vi "SetTriggerPulseWidth.vi"(8 "Error In":errorcluster, 9 "Pulse Width (sec)":dbl, 10 "Line (1-14)":u8=1 min=1 max=14 step=1, 11 "Keithley 2602 In":refnum<visa-resource-name>) -> (0 "Error Out":errorcluster, 3 "Keithley 2602 Out":refnum<visa-resource-name>)   [LabVIEW 2012, in "Keithley-2602.lvlib"]
uses:
  Keithley-2602.lvlib
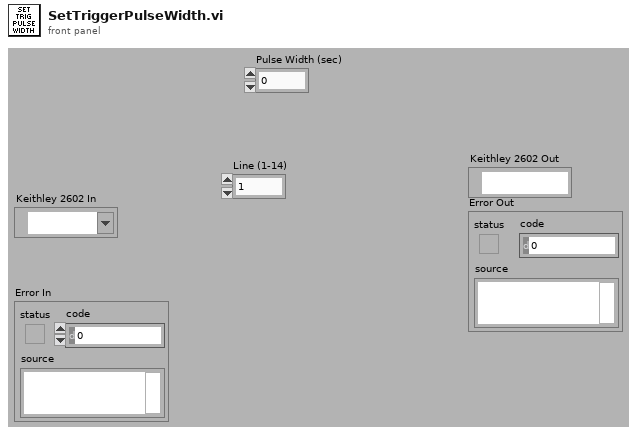
[diagram p1: front panel]
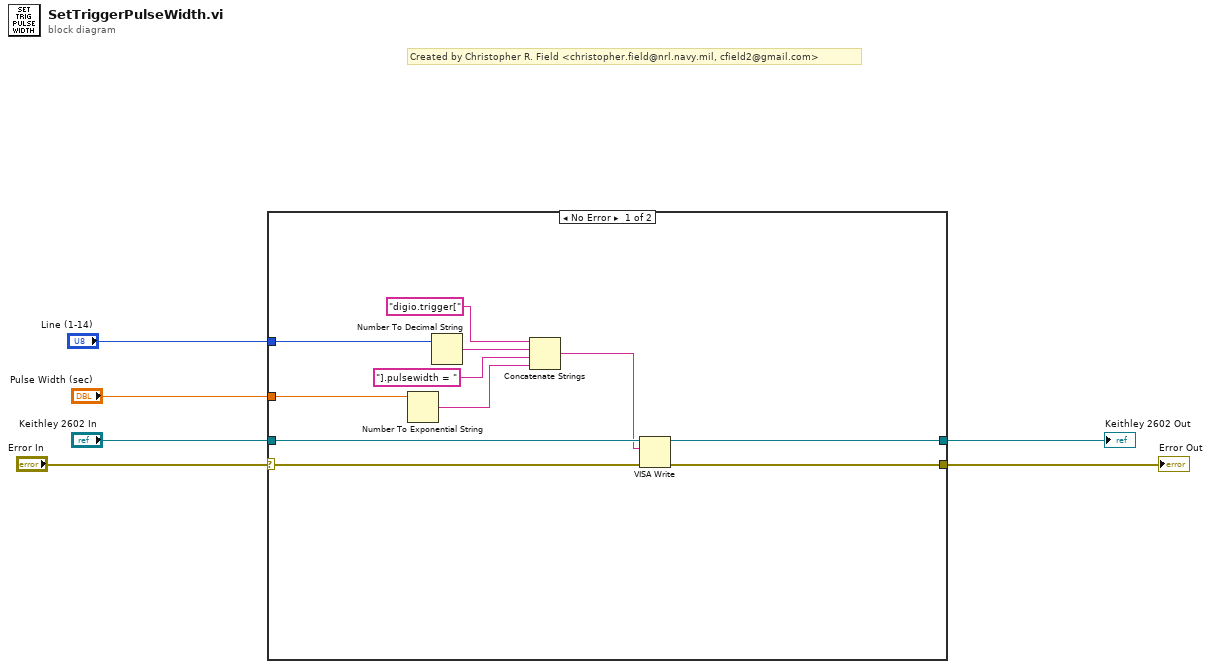
[diagram p0: block diagram]
diagram:
  # "Created by Christopher R. Field <christopher.field@nrl.navy.mil, cfield2@gmail.com>"
  n1 = case shown="No Error" "Error In" {
    selector: "Error In" -> [w7 w18]
    tunnel: "Keithley 2602 In" -> [w17 w19]
    tunnel: [w16 w19] -> w5
    tunnel: [w15 w18] -> w4
    tunnel: "Line (1-14)" -> [w14 _]
    tunnel: "Pulse Width (sec)" -> [w9 _]
    frame No Error {
      n2 = Number To Exponential String(number=w9) -> (E-format string=w8:string)  [unwired: 3 in]
      n3 = Number To Decimal String(number=w14) -> (decimal integer string=w12:string)  [unwired: 1 in]
      n4 = Concatenate Strings("digio.trigger[", w12, "].pulsewidth = ", w8) -> (w10:string)
      n5 = VISA Write(VISA resource name=w17, write buffer=w10, error in (no error)=w7) -> (VISA resource name out=w16:refnum<visa-resource-name>, error out=w15:errorcluster)  [unwired: 1 out]
    }
    frame Error {
    }
  }
  "Keithley 2602 Out" <- w5
  "Error Out" <- w4
